vi "hse-application_SystemConfiguration_ReadFile.vi"(8 "error in (no error)":errorcluster, 10 "Config File":path, 11 "hse-application in":refnum<class "hse-application.lvclass">) -> (0 "error out":errorcluster, 3 "hse-application out":refnum<class "hse-application.lvclass">)   [LabVIEW 2014, in "hse-application.lvclass"]
doc: "Reads configuration parameters from the <b>Config File</b>."
uses:
  hse-application.lvclass
  hse-application.lvclass/hse-application.ctl
  hse-configuration/hse-config-ini/hse-config-ini.lvclass
  hse-configuration/hse-config-ini/hse-config-ini_ConfigData.ctl
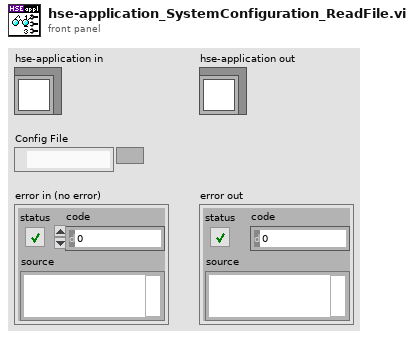
[diagram p1: front panel]
types:
  T1 = typedef "hse-config-ini.lvclass/hse-config-ini_ConfigData.ctl" = cluster{"Path to .ini file":path}
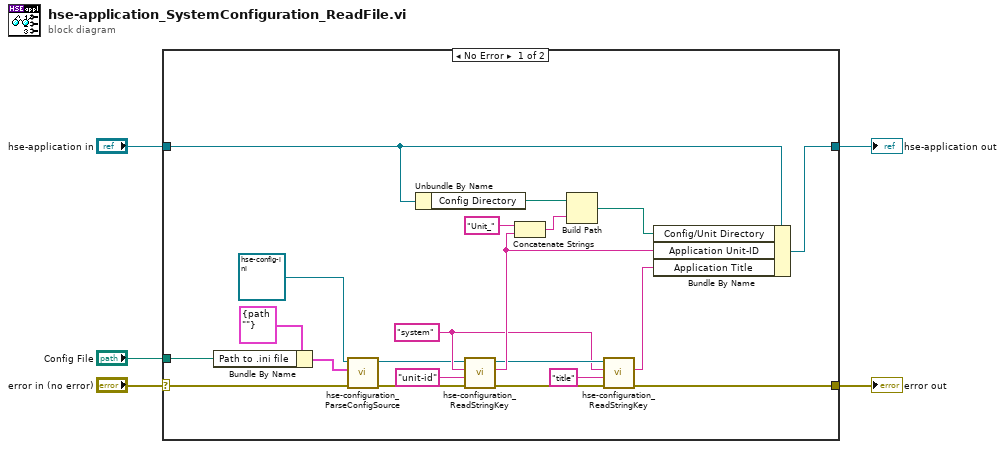
[diagram p0: block diagram]
diagram:
  n1 = case shown="No Error" "error in (no error)" {
    selector: "error in (no error)" -> [w11 w27]
    tunnel: "hse-application in" -> [w26 w28]
    tunnel: "Config File" -> [w23 _]
    tunnel: [w21 w27] -> w3
    tunnel: [w6 w28] -> w1
    frame No Error {
      w16 = "system" ("Section")
      n2 = Bundle By Name(cluster=T1 {"Path to .ini file"=path ""} ("Config Data"), "Path to .ini file"=w23) -> (w24:T1)
      n3 = call-dynamic "hse-configuration_ParseConfigSource.vi"("error in (no error)"=w11, "Config Source"=w24, "hse-config-ini in"=refnum<class "hse-config-ini.lvclass"> refnum ("hse-config-ini.lvclass")) -> ("error out"=w12:errorcluster, "hse-config-ini out"=w13:refnum<class "hse-config-ini.lvclass">)  [unwired: 7 in]
      n4 = Unbundle By Name(w26) -> ("Config Directory"=w25:path)
      n5 = call-dynamic "hse-configuration_ReadStringKey.vi"("error in (no error)"=w12, "Key"="unit-id", "Section"=w16, "hse-config-ini in"=w13) -> ("error out"=w18:errorcluster, "Value"=w19:string, "hse-config-ini out"=w17:refnum<class "hse-config-ini.lvclass">)  [unwired: 5 in]
      n6 = Concatenate Strings("Unit_" ("name or relative path"), w19) -> (w8:string)
      n7 = Build Path(base path=w25, name or relative path=w8) -> (appended path=w9:path)
      n8 = call-dynamic "hse-configuration_ReadStringKey.vi"("error in (no error)"=w18, "Key"="title", "Section"=w16, "hse-config-ini in"=w17) -> ("error out"=w21:errorcluster, "Value"=w20:string)  [unwired: 5 in, 1 out]
      n9 = Bundle By Name(cluster=w26, "Config/Unit Directory"=w9, "Application Unit-ID"=w19, "Application Title"=w20) -> (w6:refnum<class "hse-application.lvclass">)
    }
    frame Error {
    }
  }
  "error out" <- w3
  "hse-application out" <- w1
